vi "DIO 2-bit.vi"(7 "DIO0 Refnum":refnum<k21>, 9 "DIR 1:0":fxp<+,2,2> format="%04b", 10 "OUT 1:0":fxp<+,2,2> format="%04b", 11 "DIO1 Refnum":refnum<k21>) -> (2 "IN 1:0":fxp<+,2,2> format="%04b")   [LabVIEW 2017]
doc: "This VI reads 4-bit data from or writes the data to the four specified FPGA I/O items according to the direction of the data flow (<b>DIR 3:0</b>).\nFor each bit of <b>DIR 3:0</b>:\n- DIR: 1 - Write data to the corresponding bit of <b>OUT 3:0</b>\n- DIR: 0 - Read data from the corresponding bit of <b>IN 3:0</b>"
panel:
  # "This VI reads 4-bit data from or writes the data to the four specified FPGA I/O items according to the direction of the data flow (DIR 3:0).\nFor each bit of DIR 3:0:\n- DIR: 1 - Write data to the corresponding bit of OUT 3:0\n- DIR: 0 - Read data from the corresponding bit of IN 3:0"
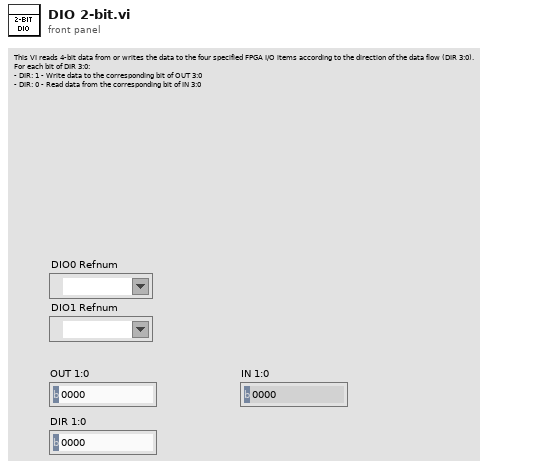
[diagram p1: front panel]
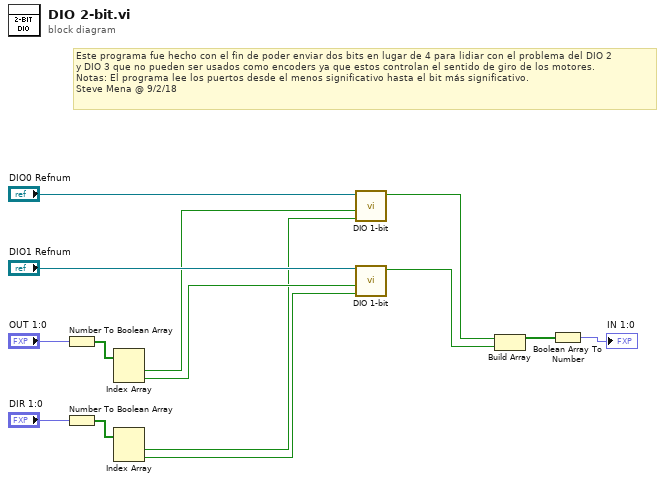
[diagram p0: block diagram]
diagram:
  # "Este programa fue hecho con el fin de poder enviar dos bits en lugar de 4 para lidiar con el problema del DIO 2\ny DIO 3 que no pueden ser usados como encoders ya que estos controlan el sentido de giro de los motores.\nNotas: El programa lee los puertos desde el menos significativo hasta el bit más significativo.\nSteve Mena @ 9/2/18"
  n1 = Number To Boolean Array(number="OUT 1:0") -> (Boolean array=w10:bool[])
  n2 = Number To Boolean Array(number="DIR 1:0") -> (Boolean array=w7:bool[])
  n3 = Index Array(array=w10) -> (element #1=w9:bool, element #2=w8:bool)  [unwired: 2 in]
  n4 = Index Array(array=w7) -> (element #1=w6:bool, element #2=w5:bool)  [unwired: 2 in]
  n5 = call "DIO 1-bit.vi"("DIR"=w6, "OUT"=w9, "DIO Refnum"="DIO0 Refnum") -> ("IN"=w4:bool)  [unwired: 8 in]
  n6 = call "DIO 1-bit.vi"("DIR"=w5, "OUT"=w8, "DIO Refnum"="DIO1 Refnum") -> ("IN"=w3:bool)  [unwired: 8 in]
  n7 = Build Array(w4, w3) -> (w2:bool[])
  n8 = Boolean Array To Number(Boolean array=w2) -> (number=→"IN 1:0":fxp<+,2,2>)
